vi "Pre_Litho_Queue.vi"(8 "error in":errorcluster, 9 "lithography_Offsets":cluster{"X":dbl, "Y":dbl}, 10 "Pattern Data":T1, 11 "Application":refnum<k7>) -> (0 "error out":errorcluster)   [LabVIEW 2020]
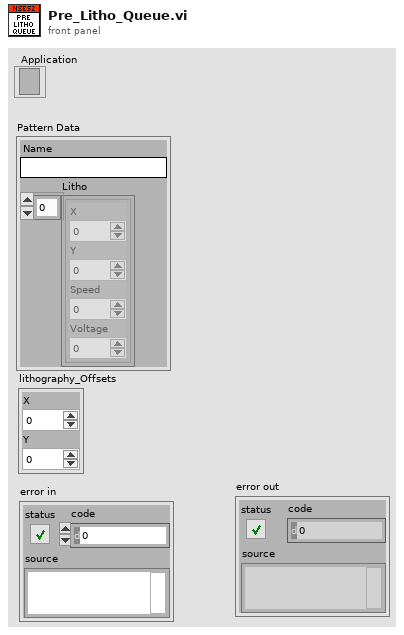
[diagram p1: front panel]
types:
  T1 = cluster{"Name":string, "Litho":cluster{"X":dbl, "Y":dbl, "Speed":dbl, "Voltage":dbl}[]}
  T2 = cluster{"X":dbl, "Y":dbl, "Speed":dbl, "Voltage":dbl}[]
  T3 = cluster{"X":dbl, "Y":dbl, "Speed":dbl, "Voltage":dbl}
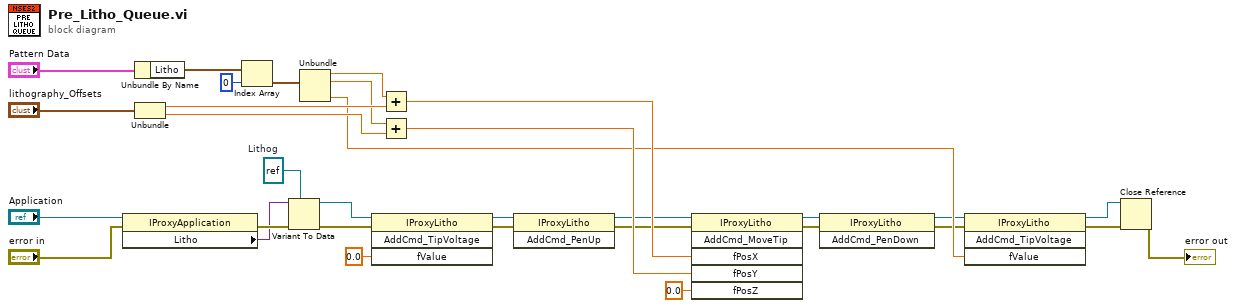
[diagram p0: block diagram]
diagram:
  w19 = refnum<k7> refnum  # Lithog
  n1 = property class="IProxyApplication"(reference="Application", error in="error in") -> (error out=w22:errorcluster, "Litho"=w21:variant)  [unwired: 1 out]
  n2 = Unbundle By Name("Pattern Data") -> ("Litho"=w31:T2)
  n3 = Unbundle("lithography_Offsets") -> ("X"=w26:dbl, "Y"=w24:dbl)
  n4 = Index Array(array=w31, index=0) -> (element=w28:T3)
  n5 = Variant To Data(error in=w22, type=w19, Variant=w21) -> (data=w18:refnum<k7>, error out=w17:errorcluster)
  n6 = Unbundle(w28) -> ("X"=w27:dbl, "Y"=w25:dbl, "Voltage"=w12:dbl)  [unwired: 1 out]
  n7 = invoke class="IProxyLitho" method="AddCmd_TipVoltage"(reference=w18, error in=w17, "fValue"=0.0) -> (reference out=w8:refnum<k7>, error out=w7:errorcluster)  [unwired: 1 in, 2 out]
  n8 = Add(x=w27, y=w26) -> (x+y=w14:dbl)
  n9 = Add(x=w25, y=w24) -> (x+y=w15:dbl)
  n10 = invoke class="IProxyLitho" method="AddCmd_PenUp"(reference=w8, error in=w7) -> (reference out=w5:refnum<k7>, error out=w6:errorcluster)  [unwired: 1 in, 1 out]
  n11 = invoke class="IProxyLitho" method="AddCmd_MoveTip"(reference=w5, error in=w6, "fPosX"=w14, "fPosY"=w15, "fPosZ"=0.0) -> (reference out=w4:refnum<k7>, error out=w3:errorcluster)  [unwired: 1 in, 4 out]
  n12 = invoke class="IProxyLitho" method="AddCmd_PenDown"(reference=w4, error in=w3) -> (reference out=w1:refnum<k7>, error out=w2:errorcluster)  [unwired: 1 in, 1 out]
  n13 = invoke class="IProxyLitho" method="AddCmd_TipVoltage"(reference=w1, error in=w2, "fValue"=w12) -> (reference out=w10:refnum<k7>, error out=w11:errorcluster)  [unwired: 1 in, 2 out]
  n14 = Close Reference(reference=w10, error in (no error)=w11) -> (error out=→"error out":errorcluster)
